vi "CRYAbout.vi"() -> ()   [LabVIEW 2013]
doc: "This VI is an adaptation of a splash screen VI developed by Steve Harrision for \"Serving Up Powerful Solutions: LabVIEW VI Server Examples\" - an article which originally appeared in the LabVIEW Technical Resource newsletter, Vol. 6 Number 4. In this example, the diagram has been simplified by replacing the original text status with a progress bar. Refer to the diagram notes and accompanying text for more details.\n\nSubscribe to the LabVIEW Technical Resource newsletter! LTR is a quarterly publication providing technical information to LabVIEW system developers.\n\nFor subscription information, back issues, and LTR VI Code Paks contact:\nLTR Publishing, Inc. \n6060 N. Central Expressway, Suite 502\nDallas, TX 75206\n(214) 706-0587\nFAX (214) 706-0506\nE-mail: subscribe@ltrpub.com\nwww.ltrpub.com"
uses:
  CRYMainGlobal.vi
panel:
  out "Message Copyright":string
  out "Message HomePage":string
  out "Message Version":string
  out "Chinese":bool
  out "English":bool
  out "Korean":bool
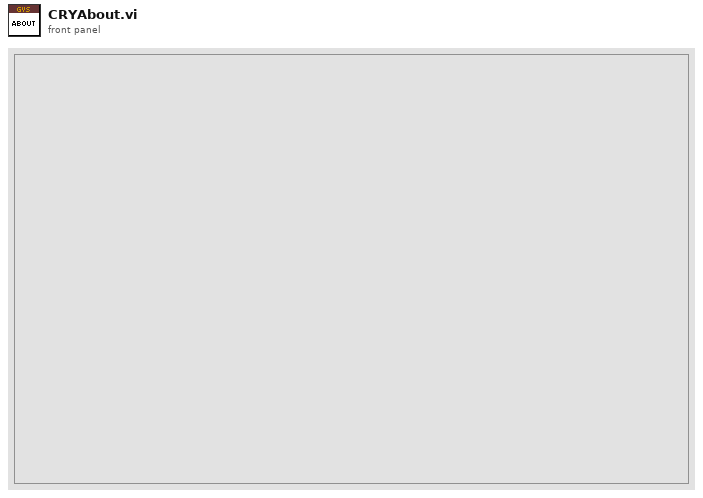
[diagram p1: front panel]
types:
  T1 = enum32{"English", "Chinese", "Korean", "Japanese", "Russian", "Chinese traditional"}
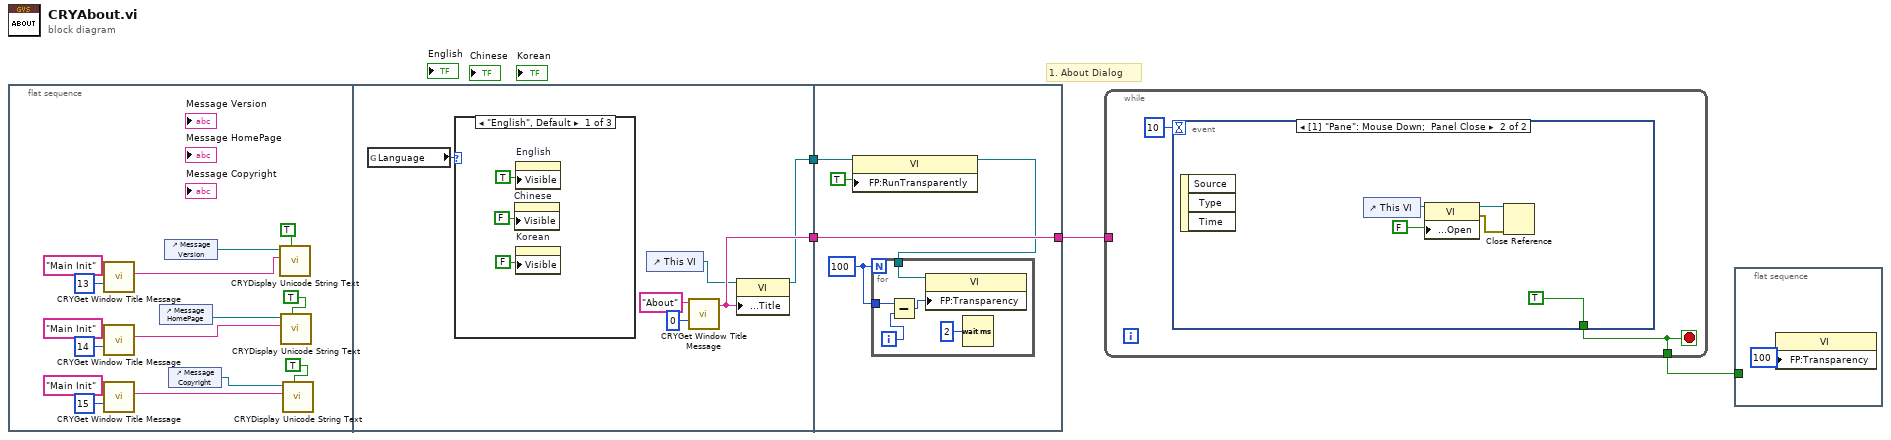
[diagram p0: block diagram]
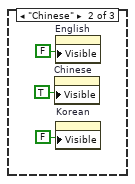
[diagram p2: hidden frame]
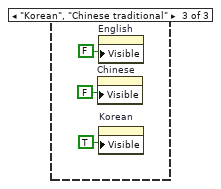
[diagram p3: hidden frame]
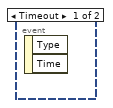
[diagram p4: hidden frame]
diagram:
  # "1. About Dialog"
  n1 = flat-sequence {
    tunnel: [w23] -> w3
    tunnel: [w20] -> w2
    tunnel: [w39] -> w4
    tunnel: w3 -> [w39]
    tunnel: w2 -> [w36]
    frame #0 {
      n2 = call "CRYGet Window Title Message.vi"("No"=13, "Kind"="Main Init") -> ("Unicode String"=w19:string)  [unwired: 4 in, 5 out]
      n3 = call "CRYGet Window Title Message.vi"("No"=14, "Kind"="Main Init") -> ("Unicode String"=w7:string)  [unwired: 4 in, 5 out]
      n4 = call "CRYGet Window Title Message.vi"("No"=15, "Kind"="Main Init") -> ("Unicode String"=w9:string)  [unwired: 4 in, 5 out]
      n5 = control-ref of="Message HomePage"() -> (w6:refnum<vi>)
      n6 = control-ref of="Message Version"() -> (w12:refnum<vi>)
      n7 = control-ref of="Message Copyright"() -> (w10:refnum<vi>)
      n8 = call "CRYDisplay Unicode String Text.vi"("Interpret as Unicode (T)"=TRUE, "String Value"=w19, "String Control Reference"=w12) -> ()  [unwired: 5 in, 2 out]
      n9 = call "CRYDisplay Unicode String Text.vi"("Interpret as Unicode (T)"=TRUE, "String Value"=w7, "String Control Reference"=w6) -> ()  [unwired: 5 in, 2 out]
      n10 = call "CRYDisplay Unicode String Text.vi"("Interpret as Unicode (T)"=TRUE, "String Value"=w9, "String Control Reference"=w10) -> ()  [unwired: 5 in, 2 out]
    }
    frame #1 {
      n11 = global read "CRYMainGlobal.vi" "Language"() -> (w22:T1)
      n12 = case shown="\"English\", Default" w22 {
        frame "English", Default {
          n13 = property on="Chinese" class="Bool (strict)"("Visible"=FALSE) -> ()  [unwired: 2 in, 2 out]
          n14 = property on="English" class="Bool (strict)"("Visible"=TRUE) -> ()  [unwired: 2 in, 2 out]
          n15 = property on="Korean" class="Bool (strict)"("Visible"=FALSE) -> ()  [unwired: 2 in, 2 out]
        }
        frame "Chinese" {
          n16 = property on="Chinese" class="Bool (strict)"("Visible"=TRUE) -> ()  [unwired: 2 in, 2 out]
          n17 = property on="English" class="Bool (strict)"("Visible"=FALSE) -> ()  [unwired: 2 in, 2 out]
          n18 = property on="Korean" class="Bool (strict)"("Visible"=FALSE) -> ()  [unwired: 2 in, 2 out]
        }
        frame "Korean", "Chinese traditional" {
          n19 = property on="Chinese" class="Bool (strict)"("Visible"=FALSE) -> ()  [unwired: 2 in, 2 out]
          n20 = property on="English" class="Bool (strict)"("Visible"=FALSE) -> ()  [unwired: 2 in, 2 out]
          n21 = property on="Korean" class="Bool (strict)"("Visible"=TRUE) -> ()  [unwired: 2 in, 2 out]
        }
      }
      n22 = control-ref of="This VI"() -> (w21:refnum<vi>)
      n23 = call "CRYGet Window Title Message.vi"("No"=0 ("Error No"), "Kind"="About") -> ("Multibyte String"=w23:string)  [unwired: 4 in, 5 out]
      n24 = property class="VI"(reference=w21, "Front Panel.Title"=w23) -> (reference out=w20:refnum<vi>)  [unwired: 1 in, 1 out]
    }
    frame #2 {
      w37 = 100
      n25 = property class="VI"(reference=w36, "FP:RunTransparently"=TRUE ("Front Panel Window:Run VI Transparently")) -> (reference out=w35:refnum<vi>)  [unwired: 1 in, 1 out]
      n26 = for {
        N: w37 -> [_]
        tunnel: w37 -> [w41]
        tunnel: w35 -> [w40]
        i -> [w43]
        n27 = Subtract(x=w41, y=w43) -> (x-y=w42:i32)
        n28 = property class="VI"(reference=w40, "FP:Transparency"=w42) -> ()  [unwired: 1 in, 2 out]
        n29 = Wait (ms)(milliseconds to wait=u32 2) -> ()  [unwired: 1 out]
      }
    }
  }
  n30 = while {
    tunnel: w4 -> [_]
    tunnel: [w46] -> w1
    stop <- w46 stop-if-true
    n31 = event shown="[1] \"Pane\": Mouse Down;  Panel Close" {
      selector: _ -> [_ _]
      dyn-events: _ -> [_ _]
      timeout: 10 -> [_ _]
      tunnel: [_ TRUE] -> w46
      event Timeout {
        n32 = event-data() -> ()  [unwired: 3 out]
      }
      event Mouse Down; Panel Close {
        n33 = event-data() -> ()  [unwired: 4 out]
        n34 = control-ref of="This VI"() -> (w47:refnum<vi>)
        n35 = property class="VI"(reference=w47, "Front Panel.Open"=FALSE ("Front Panel Window:Open")) -> (reference out=w49:refnum<vi>, error out=w48:errorcluster)  [unwired: 1 in]
        n36 = Close Reference(reference=w49, error in (no error)=w48) -> ()  [unwired: 1 out]
      }
    }
  }
  n37 = flat-sequence {
    tunnel: w1 -> [_]
    frame #0 {
      n38 = property class="VI"("FP:Transparency"=u8 100 ("Front Panel Window:Transparency")) -> ()  [unwired: 2 in, 2 out]
    }
  }
